vi "set_histogram_enabled.vi"(8 "error in (no error)":errorcluster, 11 "DisplayDL090216 in":refnum<class "DisplayDL090216.lvclass">) -> (0 "error out":errorcluster, 3 "DisplayDL090216 out":refnum<class "DisplayDL090216.lvclass">)   [LabVIEW 2010, in "DisplayDL090216.lvclass"]
uses:
  DisplayDL090216.lvclass
  DisplayDL090216.lvclass/DisplayDL090216.ctl
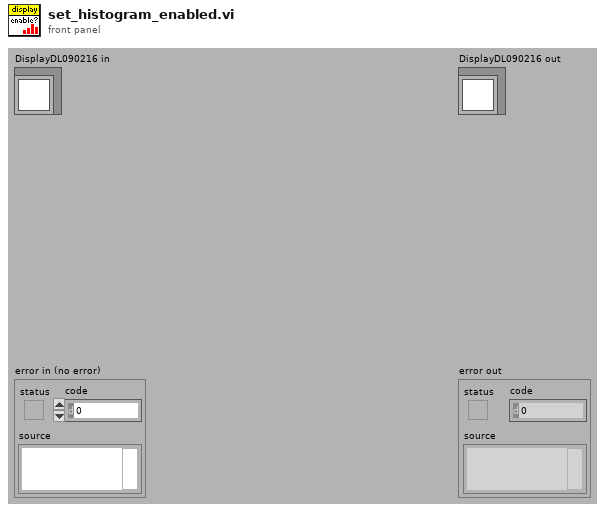
[diagram p1: front panel]
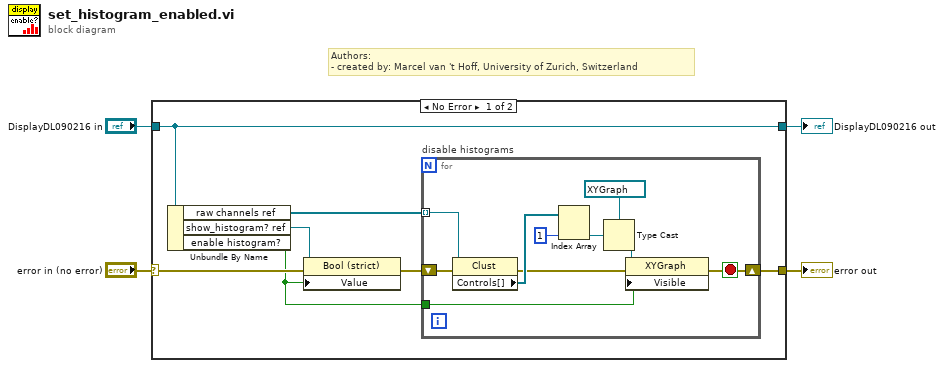
[diagram p0: block diagram]
diagram:
  # "Authors: \n- created by: Marcel van 't Hoff, University of Zurich, Switzerland"
  n1 = case shown="No Error" "error in (no error)" {
    selector: "error in (no error)" -> [w7 w23]
    tunnel: [w9 w23] -> w3
    tunnel: [w11 w22] -> w1
    tunnel: "DisplayDL090216 in" -> [w11 w22]
    frame No Error {
      n2 = Unbundle By Name(w11) -> ("raw channels ref"=w10:refnum<vi>[], "show_histogram? ref"=w8:refnum<vi>, "enable histogram?"=w5:bool)
      n3 = property class="Bool (strict)"(reference=w8, error in=w7, "Value"=w5) -> (error out=w6:errorcluster)  [unwired: 1 out]
      n4 = for "disable histograms" {
        tunnel: w10 -> [w16] mode=indexing
        shift-right: [w13] -> w9
        shift-left: w6 -> [w21]
        tunnel: w5 -> [w12]
        stop <- w13 stop-if-true
        n5 = property class="Clust"(reference=w16, error in=w21) -> (error out=w14:errorcluster, "Controls[]"=w20:refnum<vi>[])  [unwired: 1 out]
        n6 = Index Array(array=w20, index #2=1 ("index")) -> (element #2=w18:refnum<vi>)  [unwired: 1 in, 1 out]
        n7 = Type Cast(type=refnum<vi> refnum ("histogram out"), x=w18) -> (*(type *) &x=w15:refnum<vi>)
        n8 = property class="XYGraph"(reference=w15, error in=w14, "Visible"=w12) -> (error out=w13:errorcluster)  [unwired: 1 out]
      }
    }
    frame Error {
    }
  }
  "error out" <- w3
  "DisplayDL090216 out" <- w1
